vi "Console GUI (Read-Only).vi"() -> ()   [LabVIEW 2017, in "Communications Console Library.lvlib"]
uses:
  Communications Console Library.lvlib
  Typedefs/Console GUI-Program State--Enum.ctl
  Communications/Communications Library.lvlib
panel:
  out "Console Text":string
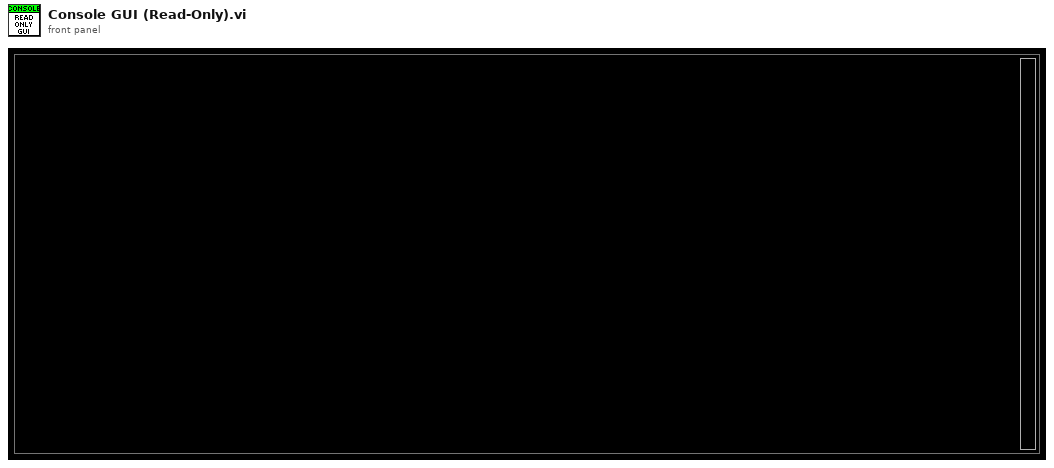
[diagram p1: front panel]
types:
  T1 = enum32{"Invalid", "Standard", "Closed", "Hidden", "Minimized", "Maximized"}
  T2 = typedef "Communications Console Library.lvlib/Console GUI-Program State--Enum.ctl" = enum16{"Load Configuration", "Send Message", "Wait", "Update GUI", "Read TCP Log File"}
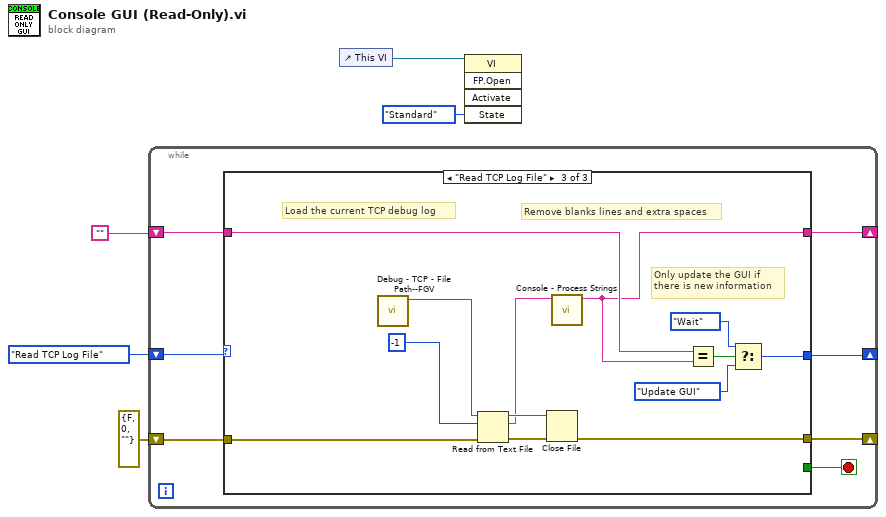
[diagram p0: block diagram]
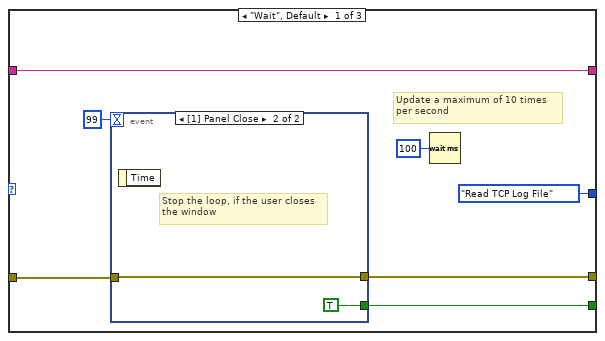
[diagram p2: hidden frame]
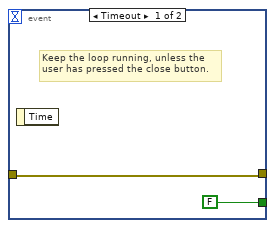
[diagram p3: hidden frame]
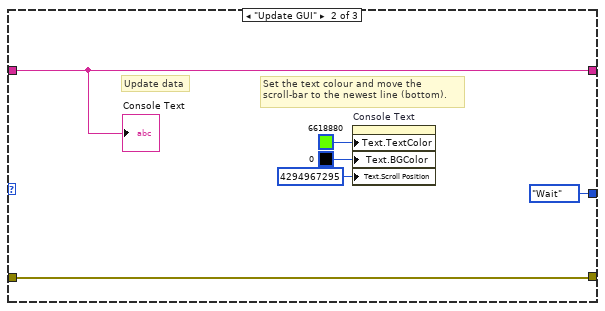
[diagram p4: hidden frame]
diagram:
  n1 = while {
    shift-right: [w12] -> _
    shift-left: "" -> [w11]
    shift-right: [w9] -> _
    shift-left: Console_GUI-Program_State--Enum."Read TCP Log File" ("Console GUI State") -> [w10]
    shift-right: [w7] -> _
    shift-left: errorcluster {"status"=FALSE, "code"=0, "source"=""} ("error out") -> [w8]
    stop <- w6 stop-if-true
    n2 = case shown="\"Read TCP Log File\"" w10 {
      tunnel: [w19 w26 w35] -> w12
      tunnel: w11 -> [w19 w26 w36]
      tunnel: [Console_GUI-Program_State--Enum."Read TCP Log File" ("Console GUI State") Console_GUI-Program_State--Enum."Wait" ("Console GUI State") w31] -> w9
      tunnel: w8 -> [w15 w24 w38]
      tunnel: [w14 w24 w37] -> w7
      tunnel: [w13 _ _] -> w6
      frame "Wait", Default {
        # "Update a maximum of 10 times\nper second"
        n3 = event shown="[1] Panel Close" {
          selector: _ -> [_ _]
          dyn-events: _ -> [_ _]
          timeout: 99 -> [_ _]
          tunnel: w15 -> [w21 w23]
          tunnel: [w21 w23] -> w14
          tunnel: [FALSE TRUE] -> w13
          event Timeout {
            # "Keep the loop running, unless the\nuser has pressed the close button."
            n4 = event-data() -> ()  [unwired: 1 in, 1 out]
          }
          event Panel Close {
            # "Stop the loop, if the user closes\nthe window"
            n5 = event-data() -> ()  [unwired: 1 in, 1 out]
          }
        }
        n6 = Wait (ms)(milliseconds to wait=u32 100) -> ()  [unwired: 1 out]
      }
      frame "Update GUI" {
        # "Update data"
        # "Set the text colour and move the \nscroll-bar to the newest line (bottom)."
        n7 = property on="Console Text" class="Str"("Text.TextColor"=u32 6618880, "Text.BGColor"=u32 0, "Text.Scroll Position"=u32 4294967295) -> ()  [unwired: 2 in, 2 out]
        "Console Text" <- w26
      }
      frame "Read TCP Log File" {
        # "Only update the GUI if\nthere is new information"
        # "Remove blanks lines and extra spaces"
        # "Load the current TCP debug log"
        n8 = call "Debug - TCP - File Path--FGV.vi"() -> ("Debug Pathname"=w30:path)  [unwired: 11 in]
        n9 = Read from Text File(file (use dialog)=w30, count=-1, error in=w38) -> (refnum out=w41:refnum<file>, text=w39:string, error out=w40:errorcluster)  [unwired: 1 in, 1 out]
        n10 = Close File(refnum=w41, error in=w40) -> (error out=w37:errorcluster)  [unwired: 1 out]
        n11 = call "Console - Process Strings.vi"("Unprocessed String"=w39) -> ("Processed String"=w35:string)  [unwired: 10 in]
        n12 = Equal?(x=w36, y=w35) -> (x = y?=w32:bool)
        n13 = Select(t=Console_GUI-Program_State--Enum."Wait" ("Console GUI State"), s=w32, f=Console_GUI-Program_State--Enum."Update GUI" ("Console GUI State")) -> (s? t:f=w31:T2)
      }
    }
  }
  n14 = control-ref of="This VI"() -> (w2:refnum<vi>)
  n15 = invoke class="VI" method="FP.Open"(reference=w2, "State"=T1."Standard") -> ()  [unwired: 3 in, 5 out]
